vi "ProcessTTRecMHT2.vi"(8 "oflcorr_in":u64, 11 "rawbits":u32) -> (0 "markercode":u32, 1 "is_marker":bool, 2 "channel":u32, 4 "oflcorr_out":u64, 5 "timetag":u64, 7 "is_photon":bool)   [LabVIEW 2023]
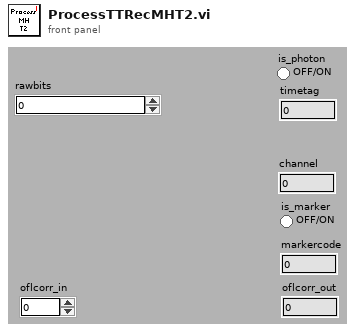
[diagram p1: front panel]
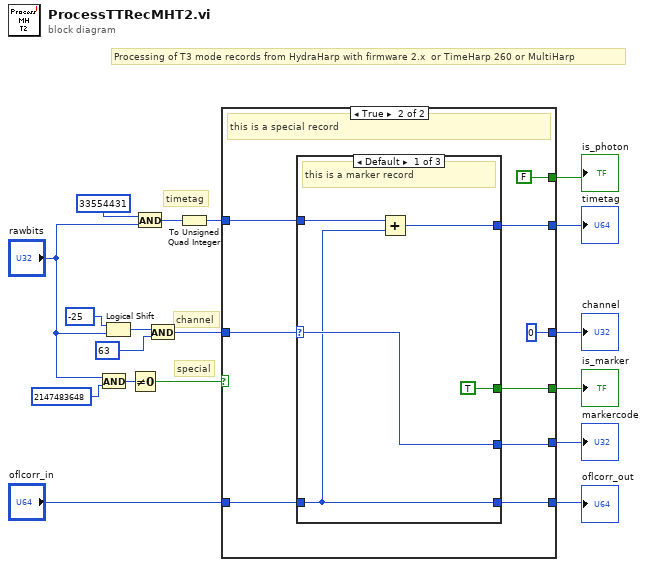
[diagram p0: block diagram]
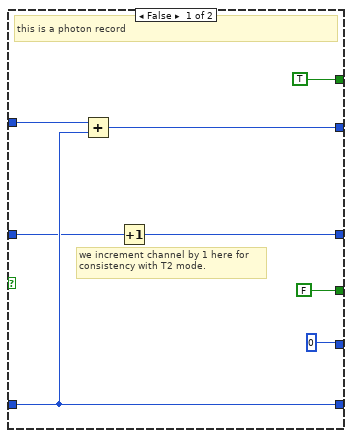
[diagram p2: hidden frame]
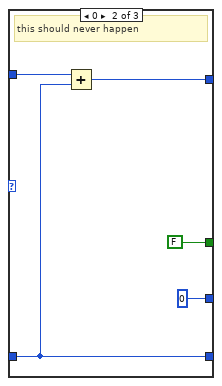
[diagram p3: hidden frame]
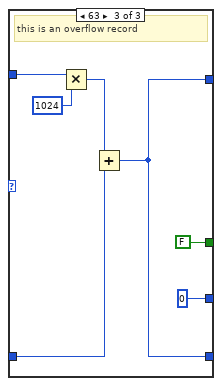
[diagram p4: hidden frame]
diagram:
  # "special"
  # "Processing of T3 mode records from HydraHarp with firmware 2.x  or TimeHarp 260 or MultiHarp"
  # "channel"
  # "timetag"
  n1 = And(x="rawbits", y=u32 2147483648 ("x")) -> (x .and. y?=w7:u32)
  n2 = Logical Shift(y=-25, x="rawbits") -> (x << y=w16:u32)
  n3 = Not Equal To 0?(x=w7) -> (x != 0?=w4:bool)
  n4 = And(x=u32 33554431, y="rawbits") -> (x .and. y?=w2:u32)
  n5 = And(x=w16, y=u32 63 ("x")) -> (x .and. y?=w3:u32)
  n6 = To Unsigned Quad Integer(1:w2) -> (0:w1:u64)
  n7 = case shown="True" w4 {
    tunnel: w1 -> [w21 w27]
    tunnel: "oflcorr_in" -> [w23 w34]
    tunnel: [w23 w33] -> w13
    tunnel: [FALSE w31] -> w11
    tunnel: [u32 0 w32] -> w12
    tunnel: [TRUE FALSE] -> w9
    tunnel: [w22 w28] -> w8
    tunnel: [w19 u32 0] -> w10
    tunnel: w3 -> [w20 w30]
    frame False {
      # "we increment channel by 1 here for\nconsistency with T2 mode."
      # "this is a photon record"
      n8 = Add(x=w21, y=w23) -> (x+y=w22:u64)
      n9 = Increment(x=w20) -> (x+1=w19:u32)
    }
    frame True {
      # "this is a special record"
      n10 = case shown="Default" w30 {
        selector: w30 -> [w39 _ _]
        tunnel: w34 -> [w37 w42 w47]
        tunnel: [w37 w42 w46] -> w33
        tunnel: [TRUE FALSE FALSE] -> w31
        tunnel: [w39 u32 0 u32 0] -> w32
        tunnel: [w36 w41 w46] -> w28
        tunnel: w27 -> [w38 w43 w50]
        frame Default {
          # "this is a marker record"
          n11 = Add(x=w38, y=w37) -> (x+y=w36:u64)
        }
        frame 0 {
          # "this should never happen"
          n12 = Add(x=w43, y=w42) -> (x+y=w41:u64)
        }
        frame 63 {
          # "this is an overflow record"
          n13 = Multiply(x=w50, y=u64 1024 ("x")) -> (x*y=w48:u64)
          n14 = Add(x=w48, y=w47) -> (x+y=w46:u64)
        }
      }
    }
  }
  "channel" <- w10
  "timetag" <- w8
  "is_photon" <- w9
  "markercode" <- w12
  "is_marker" <- w11
  "oflcorr_out" <- w13
